vi "Init_Tracks&Coord-3.vi"() -> (0 "[OUT] Tracks, Coordinates":T1)   [LabVIEW 2017]
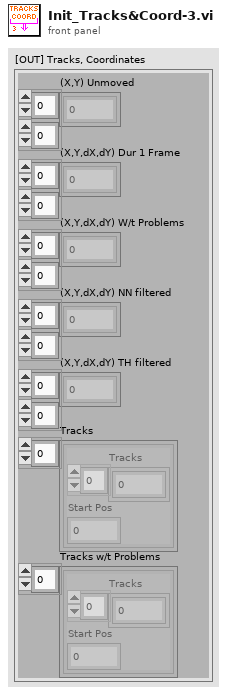
[diagram p1: front panel]
types:
  T1 = cluster{"(X,Y) Unmoved":dbl[][], "(X,Y,dX,dY) Dur 1 Frame":dbl[][], "(X,Y,dX,dY) W/t Problems":dbl[][], "(X,Y,dX,dY) NN filtered":dbl[][], "(X,Y,dX,dY) TH filtered":dbl[][], "Tracks":cluster{"Tracks":dbl[], "Start Pos":i32}[], "Tracks w/t Problems":cluster{"Tracks":dbl[], "Start Pos":i32}[]}
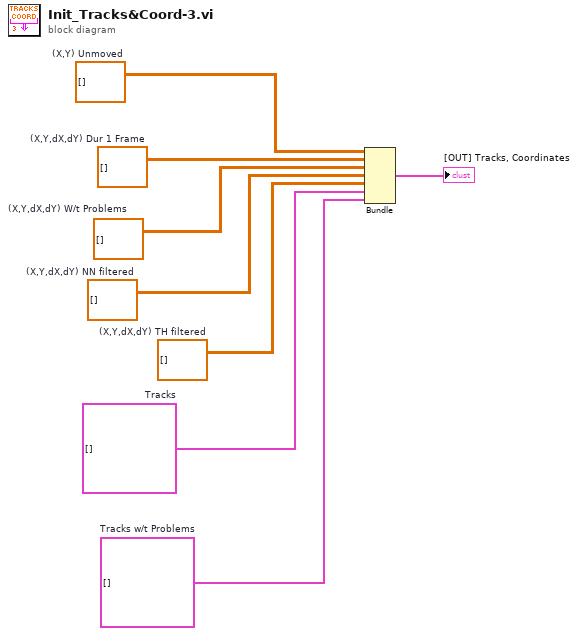
[diagram p0: block diagram]
diagram:
  w2 = cluster{"Tracks":dbl[], "Start Pos":i32}[] []  # Tracks w/t Problems
  w3 = cluster{"Tracks":dbl[], "Start Pos":i32}[] []  # Tracks
  w5 = dbl[][] []  # (X,Y,dX,dY) TH filtered
  w4 = dbl[][] []  # (X,Y,dX,dY) NN filtered
  w7 = dbl[][] []  # (X,Y,dX,dY) Dur 1 Frame
  w8 = dbl[][] []  # (X,Y) Unmoved
  w6 = dbl[][] []  # (X,Y,dX,dY) W/t Problems
  n1 = Bundle("(X,Y) Unmoved"=w8, "(X,Y,dX,dY) Dur 1 Frame"=w7, "(X,Y,dX,dY) W/t Problems"=w6, "(X,Y,dX,dY) NN filtered"=w4, "(X,Y,dX,dY) TH filtered"=w5, "Tracks"=w3, "Tracks w/t Problems"=w2) -> (→"[OUT] Tracks, Coordinates":T1)  [unwired: 1 in]
